vi "DTC.Descriptor.Override.vi"(10 "Byte Lengths":T2, 11 "Descriptor in":T1={"DTC Byte Length"=2, "Status Byte Length"=1, "Add Data Byte Length"=0, "Byte Order"=enum."Motorola"}) -> (3 "Descriptor out":T1={"DTC Byte Length"=2, "Status Byte Length"=1, "Add Data Byte Length"=0, "Byte Order"=enum."Motorola"})   [LabVIEW 2019, in "Diagnostics Addon Engine.lvlib"]
uses:
  Diagnostics Addon Engine.lvlib
  Addon Shared/Types/DTC.Descriptor.Override.ctl
  Addon Shared/Types/DTC.Descriptor.ctl
  Addon Shared/Diagnostics Addon Shared.lvlib
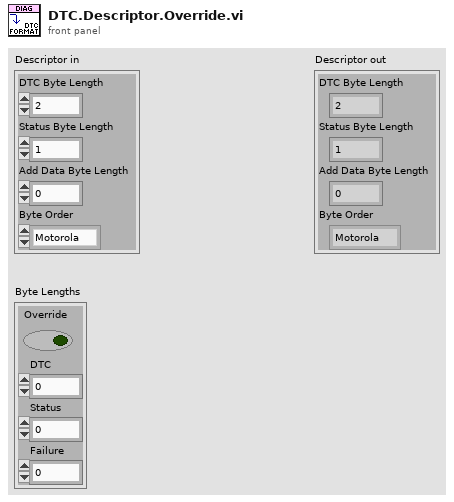
[diagram p1: front panel]
types:
  T1 = typedef "Diagnostics Addon Shared.lvlib/DTC.Descriptor.ctl" = cluster{"DTC Byte Length":i32, "Status Byte Length":i32, "Add Data Byte Length":i32, "Byte Order":enum16{"Motorola", "Intel"}}
  T2 = typedef "Diagnostics Addon Shared.lvlib/DTC.Descriptor.Override.ctl" = cluster{"Override":bool, "DTC":u32, "Status":u32, "Failure":u32}
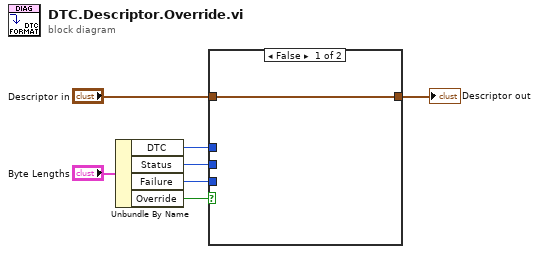
[diagram p0: block diagram]
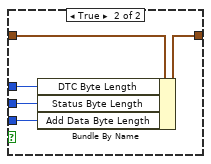
[diagram p2: hidden frame]
diagram:
  n1 = Unbundle By Name("Byte Lengths") -> ("DTC"=w3:u32, "Status"=w2:u32, "Failure"=w1:u32, "Override"=w6:bool)
  n2 = case shown="False" w6 {
    tunnel: "Descriptor in" -> [w8 w13]
    tunnel: [w8 w9] -> w4
    tunnel: w3 -> [_ w12]
    tunnel: w2 -> [_ w11]
    tunnel: w1 -> [_ w10]
    frame False {
    }
    frame True {
      n3 = Bundle By Name(cluster=w13, "DTC Byte Length"=w12, "Status Byte Length"=w11, "Add Data Byte Length"=w10) -> (w9:T1)
    }
  }
  "Descriptor out" <- w4
